vi "FinalProject.vi"() -> ()   [LabVIEW 2016]
uses:
  <vilib>/DAQmx/read.llb/DAQmx Read (Digital Bool 1Line 1Point).vi
  <vilib>/DAQmx/write.llb/DAQmx Write (Digital Bool 1Line 1Point).vi
  <vilib>/DAQmx/create/channels.llb/DAQmx Create Channel (DI-Digital Input).vi
  <vilib>/DAQmx/create/channels.llb/DAQmx Create Channel (DO-Digital Output).vi
  <vilib>/Utility/file.llb/Write Delimited Spreadsheet (DBL).vi
  <vilib>/DAQmx/miscellaneous.llb/DAQmx Fill In Error Info.vi
  <vilib>/ptbypt/NI_PtbyPt.lvlib
panel:
  in  "Stop Button":bool
  in  "Start Button":bool
  out "new file path (Not A Path if cancelled)":path
  out "BELT":bool=TRUE
  out "CHAIN":bool=TRUE
  out "Stop":bool
  out "Start":bool=TRUE
  out "Asem":i32
  out "Temp.1 2":i32
  out "Temp.1":i32
  out "Final Plastic":dbl(slide) scale=0.0..12.0 scale format="%#_12g"
  out "Final Metal":dbl(slide) scale=0.0..12.0 scale format="%#_12g"
  out "Metal detector on QA Rejector":bool
  out "temp.":i32
  out "Final Assembly":i32(knob) scale=0.0..12.0 scale format="%#.12g"
  out "Plastic rejection temp":dbl
  out "Metal rejected temp":dbl
  out "leave assembble":i32
  out "Assembly and Laser":i32
  out "Assembly":i32
  out "Numeric 5":i32
  out "Numeric 4":i32
  in  "stop 2":bool
  out "Assembly Count":u32
  out "Numeric 3":i32
  out "Numeric 2":u32
  out "metal clear 1":u32
  out "Metal Count 2":u32
  out "Metal count temp 2":dbl
  out "Numeric":i32
  out "Assemble Temp":u32
  out "Proximity (BELT)":bool
  in  "QA Rejector (plastic/metal)":bool
  out "Plastic in Chute":dbl(knob) scale=0.0..6.0 scale format="%#_10g"
  out "Metal Detector (CHAIN)":bool
  out "Proximity (CHAIN)":bool
  out "Laser (BELT)":bool
  out "Metal Detector (BELT)":bool
  out "Complete Assembly\n Detector (False when assem is there)":bool
  out "Rotary Proximity":bool
  in  "Rotary Motor":bool
  in  "Kicker (CHAIN)":bool
  in  "stop":bool
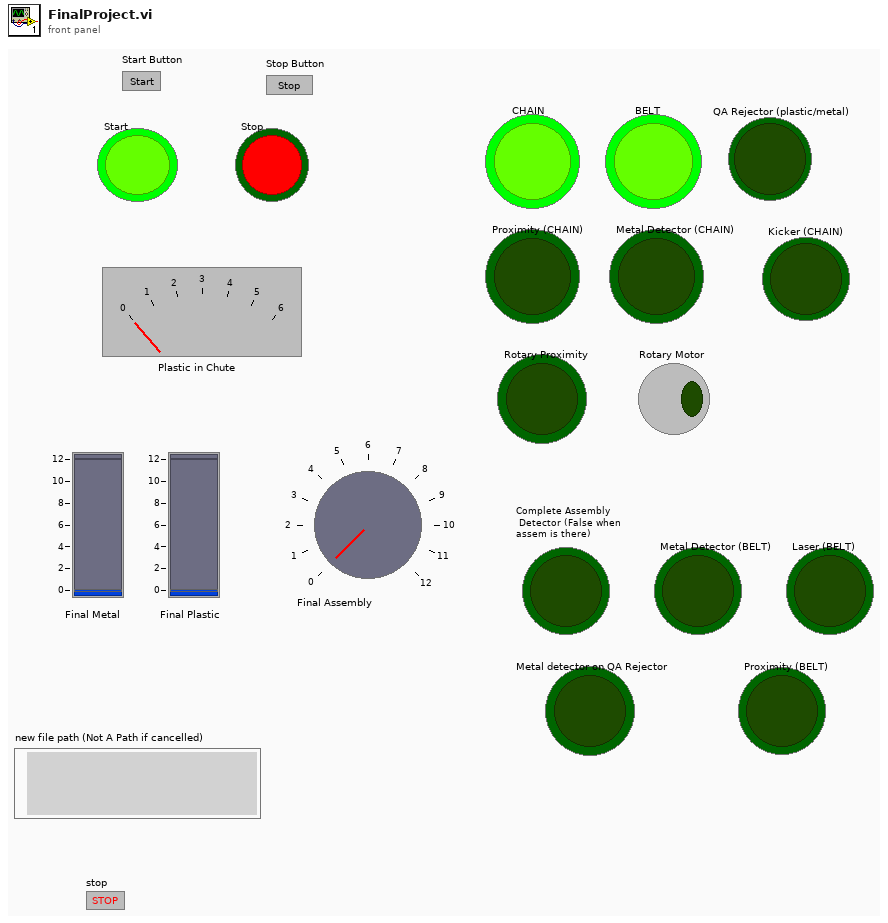
[diagram p1: front panel]
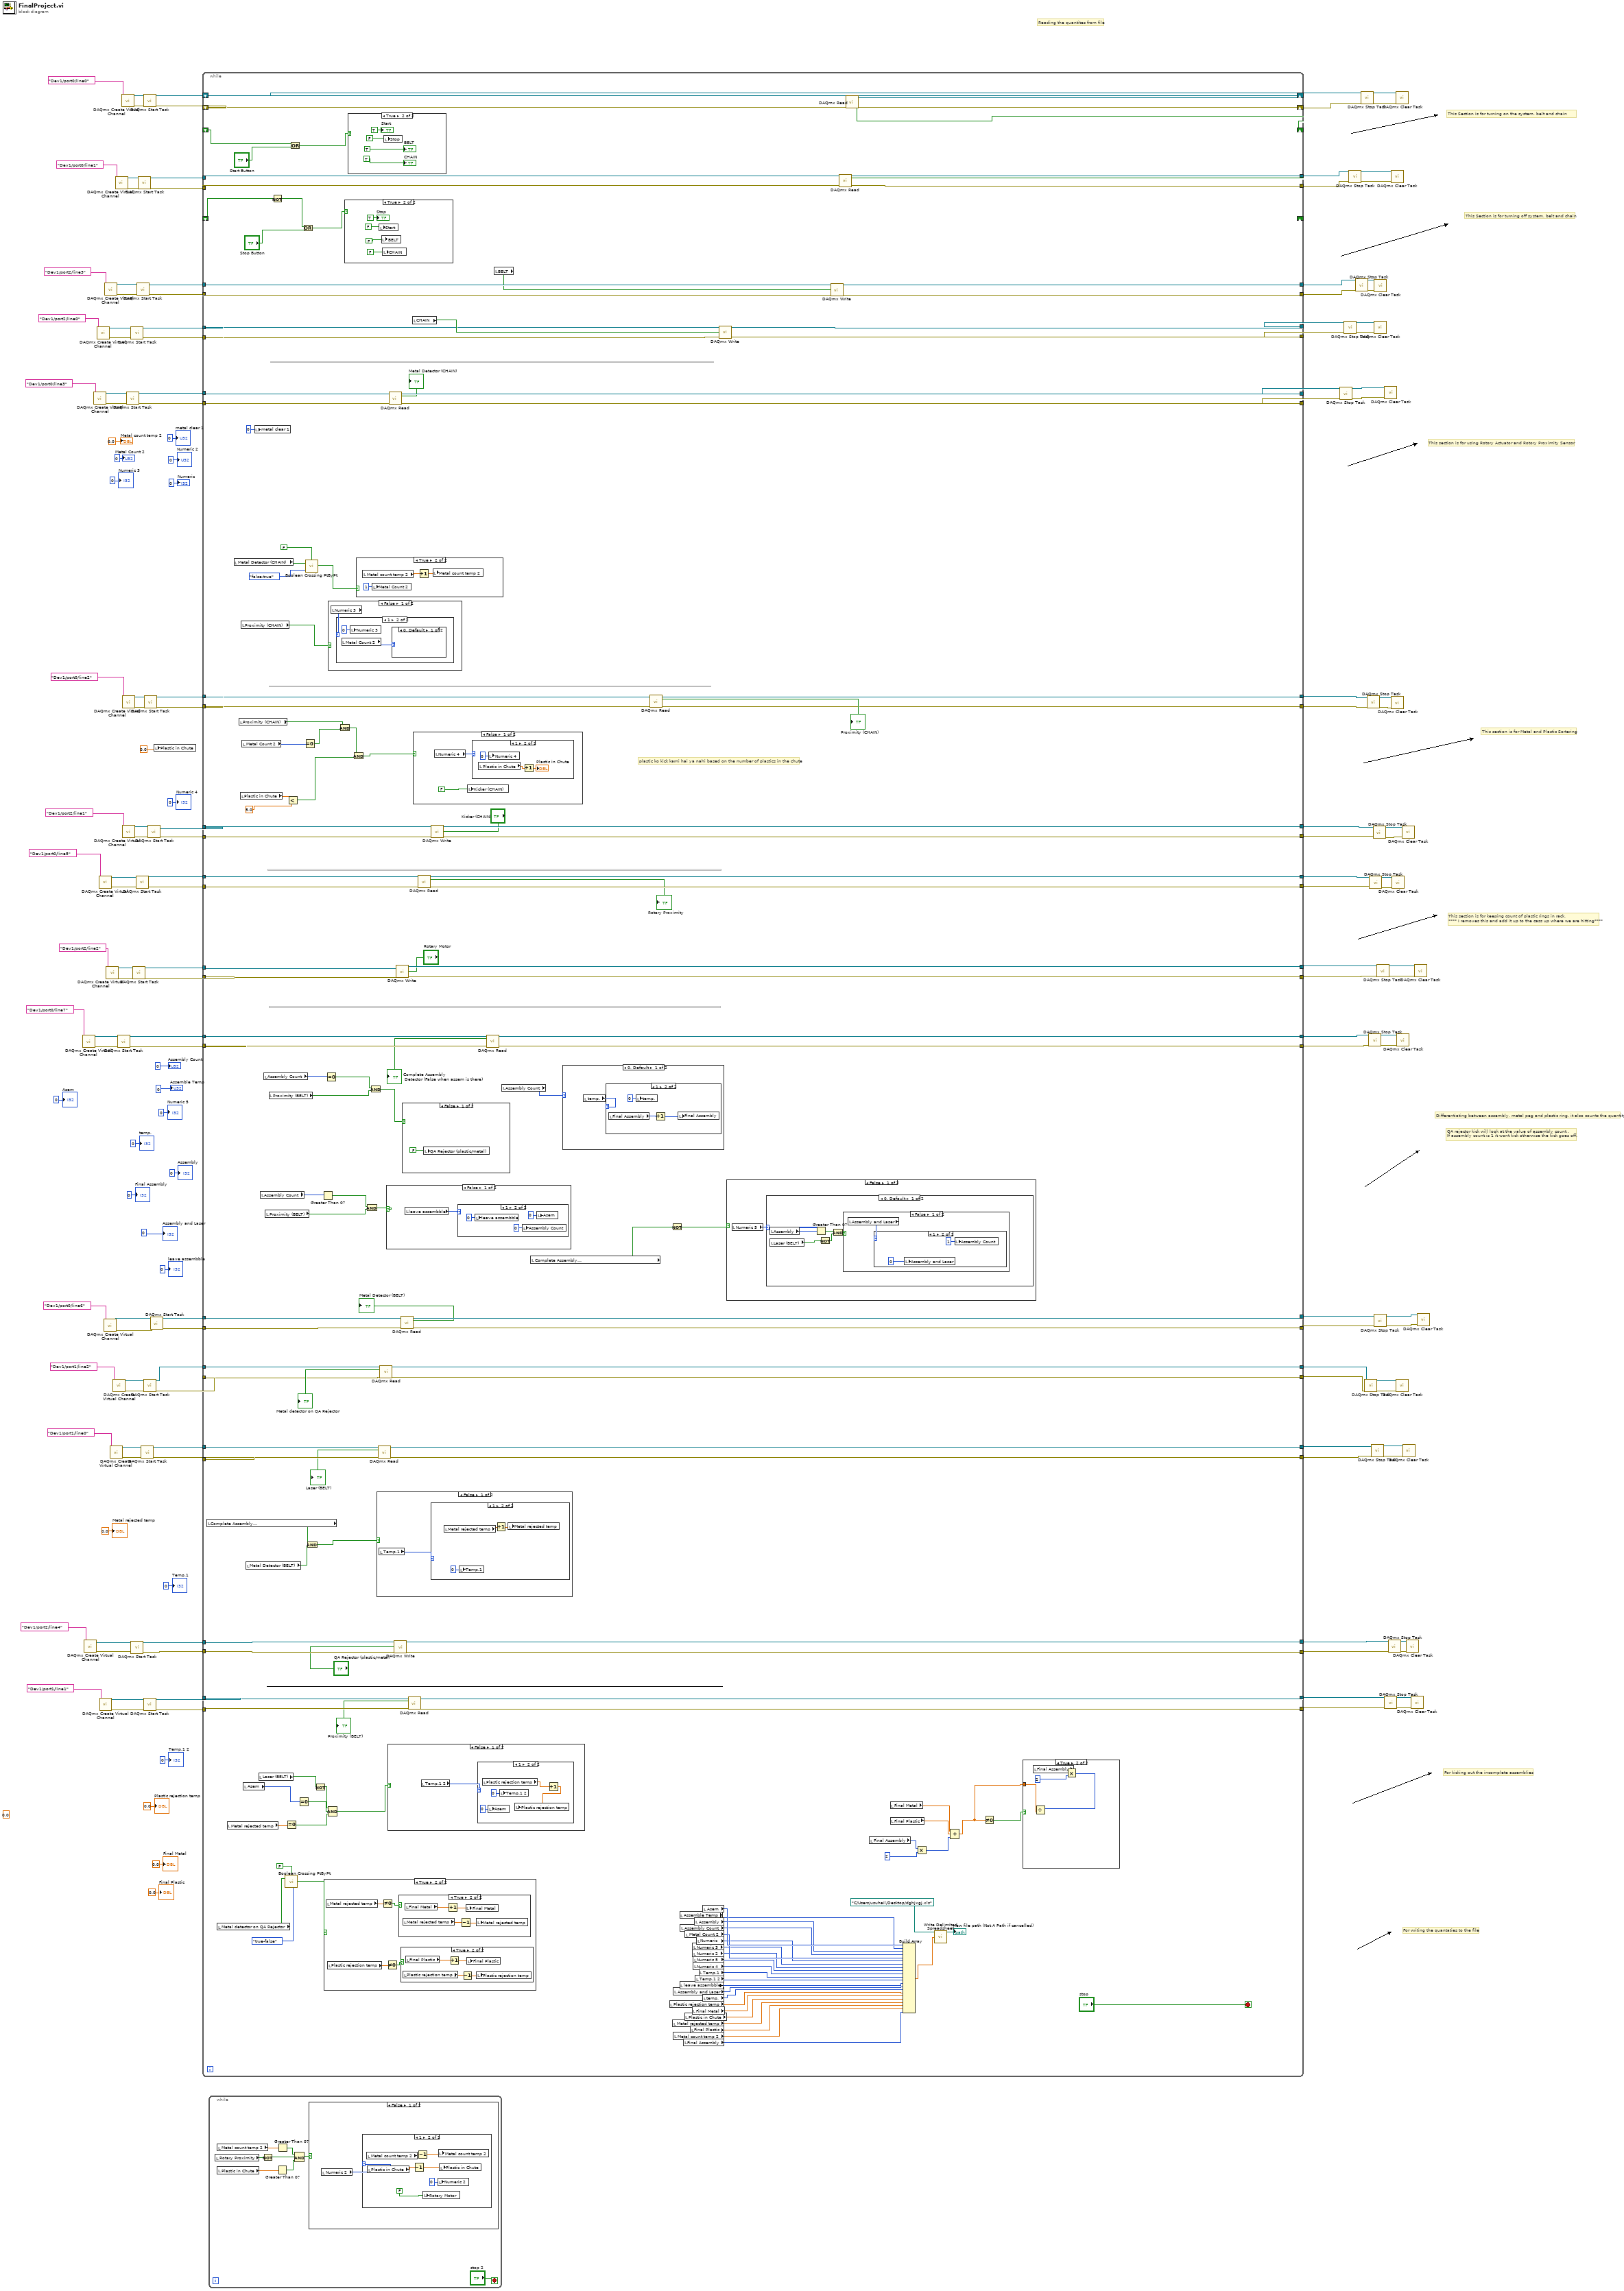
[diagram p0: block diagram]
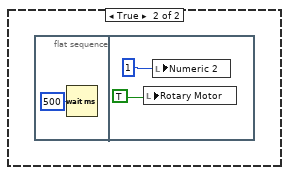
[diagram p3: hidden frame]
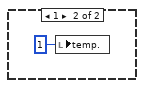
[diagram p9: hidden frame]
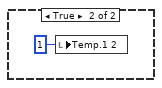
[diagram p11: hidden frame]
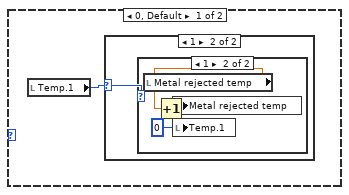
[diagram p12: hidden frame]
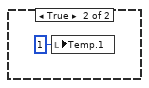
[diagram p15: hidden frame]
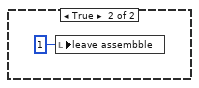
[diagram p17: hidden frame]
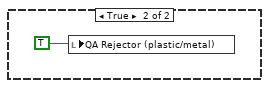
[diagram p18: hidden frame]
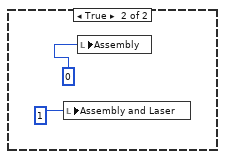
[diagram p20: hidden frame]
diagram:
  (unwired) 0.0
  # "QA rejector kick will look at the value of assembly count .\nIf assembly count is 1 it wont kick otherwise the kick goes off."
  # "Reading the quantites from file"
  # "For writing the quantaties to the file"
  # "For kicking out the incomplete assemblies"
  # "Differentiating between assembly, metal peg and plastic ring. it also counts the quantity"
  # "This section is for keeping count of plastic rings in rack. \n**** I removes this and add it up to the cass up where we are hitting****"
  # "This section is for using Rotory Actuator and Rotory Proximity Sensor"
  # "This Section is for turning off system, belt and chain"
  # "This Section is for turning on the system, belt and chain"
  # "This section is for Metal and Plastic Sortering"
  n1 = call-poly <vilib>:"DAQmx Create Virtual Channel.vi"("lines"=tag "Dev1/port0/line7") -> ("task out"=w76:refnum<k21>, "error out"=w75:errorcluster)  [unwired: 13 in]
  n2 = call-poly <vilib>:"DAQmx Create Virtual Channel.vi"("lines"=tag "Dev1/port2/line4") -> ("task out"=w48:refnum<k21>, "error out"=w47:errorcluster)  [unwired: 13 in]
  n3 = call-poly <vilib>:"DAQmx Create Virtual Channel.vi"("lines"=tag "Dev1/port0/line3") -> ("task out"=w119:refnum<k21>, "error out"=w118:errorcluster)  [unwired: 13 in]
  n4 = call-poly <vilib>:"DAQmx Create Virtual Channel.vi"("lines"=tag "Dev1/port2/line0") -> ("task out"=w128:refnum<k21>, "error out"=w127:errorcluster)  [unwired: 13 in]
  n5 = call-poly <vilib>:"DAQmx Create Virtual Channel.vi"("lines"=tag "Dev1/port0/line5") -> ("task out"=w94:refnum<k21>, "error out"=w93:errorcluster)  [unwired: 13 in]
  n6 = call-poly <vilib>:"DAQmx Create Virtual Channel.vi"("lines"=tag "Dev1/port1/line1") -> ("task out"=w39:refnum<k21>, "error out"=w38:errorcluster)  [unwired: 13 in]
  n7 = call-poly <vilib>:"DAQmx Create Virtual Channel.vi"("lines"=tag "Dev1/port0/line6") -> ("task out"=w69:refnum<k21>, "error out"=w68:errorcluster)  [unwired: 13 in]
  n8 = call-poly <vilib>:"DAQmx Create Virtual Channel.vi"("lines"=tag "Dev1/port2/line3") -> ("task out"=w137:refnum<k21>, "error out"=w136:errorcluster)  [unwired: 13 in]
  n9 = call-poly <vilib>:"DAQmx Create Virtual Channel.vi"("lines"=tag "Dev1/port2/line2") -> ("task out"=w85:refnum<k21>, "error out"=w84:errorcluster)  [unwired: 13 in]
  n10 = call-poly <vilib>:"DAQmx Create Virtual Channel.vi"("lines"=tag "Dev1/port1/line0") -> ("task out"=w58:refnum<k21>, "error out"=w57:errorcluster)  [unwired: 13 in]
  n11 = call-poly <vilib>:"DAQmx Create Virtual Channel.vi"("lines"=tag "Dev1/port1/line2") -> ("task out"=w13:refnum<k21>, "error out"=w14:errorcluster)  [unwired: 13 in]
  n12 = call-poly <vilib>:"DAQmx Create Virtual Channel.vi"("lines"=tag "Dev1/port0/line1") -> ("task out"=w149:refnum<k21>, "error out"=w147:errorcluster)  [unwired: 13 in]
  n13 = call <vilib>:"DAQmx Start Task.vi"("task/channels in"=w76, "error in"=w75) -> ("task out"=w74:refnum<k21>, "error out"=w73:errorcluster)  [unwired: 12 in]
  n14 = call-poly <vilib>:"DAQmx Create Virtual Channel.vi"("lines"=tag "Dev1/port0/line0") -> ("task out"=w158:refnum<k21>, "error out"=w154:errorcluster)  [unwired: 13 in]
  n15 = call-poly <vilib>:"DAQmx Create Virtual Channel.vi"("lines"=tag "Dev1/port0/line2") -> ("task out"=w111:refnum<k21>, "error out"=w110:errorcluster)  [unwired: 13 in]
  n16 = call-poly <vilib>:"DAQmx Create Virtual Channel.vi"("lines"=tag "Dev1/port2/line1") -> ("task out"=w103:refnum<k21>, "error out"=w102:errorcluster)  [unwired: 13 in]
  n17 = call <vilib>:"DAQmx Start Task.vi"("task/channels in"=w119, "error in"=w118) -> ("task out"=w116:refnum<k21>, "error out"=w115:errorcluster)  [unwired: 12 in]
  n18 = call <vilib>:"DAQmx Start Task.vi"("task/channels in"=w128, "error in"=w127) -> ("task out"=w126:refnum<k21>, "error out"=w125:errorcluster)  [unwired: 12 in]
  n19 = call <vilib>:"DAQmx Start Task.vi"("task/channels in"=w48, "error in"=w47) -> ("task out"=w44:refnum<k21>, "error out"=w43:errorcluster)  [unwired: 12 in]
  n20 = call <vilib>:"DAQmx Start Task.vi"("task/channels in"=w85, "error in"=w84) -> ("task out"=w83:refnum<k21>, "error out"=w82:errorcluster)  [unwired: 12 in]
  n21 = call <vilib>:"DAQmx Start Task.vi"("task/channels in"=w94, "error in"=w93) -> ("task out"=w92:refnum<k21>, "error out"=w91:errorcluster)  [unwired: 12 in]
  n22 = call <vilib>:"DAQmx Start Task.vi"("task/channels in"=w137, "error in"=w136) -> ("task out"=w135:refnum<k21>, "error out"=w134:errorcluster)  [unwired: 12 in]
  n23 = call <vilib>:"DAQmx Start Task.vi"("task/channels in"=w149, "error in"=w147) -> ("task out"=w144:refnum<k21>, "error out"=w143:errorcluster)  [unwired: 12 in]
  n24 = call <vilib>:"DAQmx Start Task.vi"("task/channels in"=w58, "error in"=w57) -> ("task out"=w56:refnum<k21>, "error out"=w55:errorcluster)  [unwired: 12 in]
  n25 = call <vilib>:"DAQmx Start Task.vi"("task/channels in"=w158, "error in"=w154) -> ("task out"=w157:refnum<k21>, "error out"=w153:errorcluster)  [unwired: 12 in]
  n26 = call <vilib>:"DAQmx Start Task.vi"("task/channels in"=w39, "error in"=w38) -> ("task out"=w37:refnum<k21>, "error out"=w36:errorcluster)  [unwired: 12 in]
  n27 = call <vilib>:"DAQmx Start Task.vi"("task/channels in"=w13, "error in"=w14) -> ("task out"=w11:refnum<k21>, "error out"=w10:errorcluster)  [unwired: 12 in]
  n28 = call <vilib>:"DAQmx Start Task.vi"("task/channels in"=w111, "error in"=w110) -> ("task out"=w109:refnum<k21>, "error out"=w108:errorcluster)  [unwired: 12 in]
  n29 = call <vilib>:"DAQmx Start Task.vi"("task/channels in"=w103, "error in"=w102) -> ("task out"=w101:refnum<k21>, "error out"=w100:errorcluster)  [unwired: 12 in]
  n30 = call <vilib>:"DAQmx Start Task.vi"("task/channels in"=w69, "error in"=w68) -> ("task out"=w65:refnum<k21>, "error out"=w60:errorcluster)  [unwired: 12 in]
  n31 = local write "Plastic in Chute"(0.0) -> ()
  n32 = while {
    shift-right: [w311] -> w156
    shift-left: w157 -> [w312]
    shift-right: [w309] -> w152
    shift-left: w153 -> [w310]
    shift-right: [w307] -> _
    shift-left: _ -> [w164]
    tunnel: w144 -> [w306]
    tunnel: w143 -> [w305]
    tunnel: [w304] -> w142
    tunnel: [w303] -> w141
    shift-right: [w302] -> _
    shift-left: _ -> [w301]
    tunnel: w135 -> [w297]
    tunnel: w134 -> [w300]
    tunnel: [w299] -> w133
    tunnel: [w298] -> w132
    tunnel: w126 -> [w293]
    tunnel: w125 -> [w294]
    tunnel: [w292] -> w124
    tunnel: [w291] -> w123
    tunnel: [w285] -> w117
    tunnel: w116 -> [w287]
    tunnel: w115 -> [w286]
    tunnel: w109 -> [w290]
    tunnel: w108 -> [w289]
    tunnel: [w288] -> w106
    tunnel: [w228] -> w107
    tunnel: [w231] -> w105
    tunnel: w101 -> [w284]
    tunnel: w100 -> [w283]
    tunnel: [w282] -> w99
    tunnel: [w281] -> w98
    tunnel: w92 -> [w280]
    tunnel: w91 -> [w279]
    tunnel: [w278] -> w88
    tunnel: [w277] -> w87
    tunnel: w83 -> [w276]
    tunnel: w82 -> [w275]
    tunnel: [w274] -> w79
    tunnel: [w273] -> w78
    tunnel: w74 -> [w271]
    tunnel: w73 -> [w268]
    tunnel: w65 -> [w267]
    tunnel: [w265] -> w64
    tunnel: [w264] -> w63
    tunnel: [w270] -> w62
    tunnel: [w269] -> w61
    tunnel: w60 -> [w266]
    tunnel: w56 -> [w259]
    tunnel: w55 -> [w258]
    tunnel: [w257] -> w52
    tunnel: [w256] -> w51
    tunnel: w44 -> [w243]
    tunnel: w43 -> [w240]
    tunnel: [w242] -> w42
    tunnel: [w241] -> w41
    tunnel: w37 -> [w238]
    tunnel: w36 -> [w237]
    tunnel: [w236] -> w33
    tunnel: [w235] -> w32
    tunnel: w11 -> [w214]
    tunnel: w10 -> [w213]
    tunnel: [w212] -> w7
    tunnel: [w211] -> w6
    stop <- "stop" stop-if-true
    # "plastic ko kick karni hai ya nahi based on the number of plastics in the chute"
    n33 = local read "Complete Assembly\n Detector (False when assem is there)"() -> (w206:bool)
    n34 = local read "Metal detector on QA Rejector"() -> (w209:bool)
    n35 = local read "Metal rejected temp"() -> (w203:dbl)
    n36 = local read "Metal Detector (CHAIN)"() -> (w233:bool)
    n37 = local read "Proximity (CHAIN)"() -> (w250:bool)
    n38 = local read "Plastic in Chute"() -> (w247:dbl)
    n39 = local read "Proximity (CHAIN)"() -> (w229:bool)
    n40 = local read "Metal Count 2"() -> (w230:u32)
    n41 = local read "Asem"() -> (w197:i32)
    n42 = local read "Metal Detector (BELT)"() -> (w205:bool)
    n43 = local write "metal clear 1"(u32 0 ("metal clear 1")) -> ()
    n44 = local read "Laser (BELT)"() -> (w201:bool)
    n45 = local read "Assembly Count"() -> (w219:u32)
    n46 = local read "Assembly Count"() -> (w226:u32)
    n47 = local read "Proximity (BELT)"() -> (w221:bool)
    n48 = local read "Proximity (BELT)"() -> (w224:bool)
    n49 = Not(x=w301) -> (.not. x?=w160:bool)
    n50 = call <vilib>:"Boolean Crossing PtByPt.vi"("initialize"=FALSE, "direction"=enum16{"either", "false-true", "true-false"}."true-false", "input"=w209) -> ("crossing"=w208:bool)
    n51 = Equal To 0?(x=w203) -> (x = 0?=w202:bool)
    n52 = Less?(x=w247, y=5.0) -> (x < y?=w244:bool)
    n53 = Or(x=w164, y="Start Button") -> (x .or. y?=w162:bool)
    n54 = Equal To 0?(x=w197) -> (x = 0?=w199:bool)
    n55 = Or(x=w160, y="Stop Button") -> (x .or. y?=w159:bool)
    n56 = Equal To 0?(x=w230) -> (x = 0?=w249:bool)
    n57 = call <vilib>:"Boolean Crossing PtByPt.vi"("initialize"=FALSE, "direction"=enum16{"either", "false-true", "true-false"}."false-true", "input"=w233) -> ("crossing"=w251:bool)
    n58 = And(x=w206, y=w205) -> (x .and. y?=w204:bool)
    n59 = Not(x=w201) -> (.not. x?=w200:bool)
    n60 = Greater Than 0?(x=w219) -> (x > 0?=w220:bool)
    n61 = case shown="True" w208 {
      frame False {
      }
      frame True {
        n62 = local read "Metal rejected temp"() -> (w320:dbl)
        n63 = local read "Plastic rejection temp"() -> (w318:dbl)
        n64 = Not Equal To 0?(x=w320) -> (x != 0?=w319:bool)
        n65 = Not Equal To 0?(x=w318) -> (x != 0?=w317:bool)
        n66 = case shown="True" w319 {
          frame False {
          }
          frame True {
            n67 = local read "Metal rejected temp"() -> (w326:dbl)
            n68 = local read "Final Metal"() -> (w327:dbl)
            n69 = Increment(x=w327) -> (x+1=w328:dbl)
            n70 = Decrement(x=w326) -> (x-1=w325:dbl)
            n71 = local write "Final Metal"(w328) -> ()
            n72 = local write "Metal rejected temp"(w325) -> ()
          }
        }
        n73 = case shown="True" w317 {
          frame False {
          }
          frame True {
            n74 = local read "Plastic rejection temp"() -> (w323:dbl)
            n75 = local read "Final Plastic"() -> (w322:dbl)
            n76 = Increment(x=w322) -> (x+1=w321:dbl)
            n77 = Decrement(x=w323) -> (x-1=w324:dbl)
            n78 = local write "Final Plastic"(w321) -> ()
            n79 = local write "Plastic rejection temp"(w324) -> ()
          }
        }
      }
    }
    n80 = Equal To 0?(x=w226) -> (x = 0?=w225:bool)
    n81 = case shown="False" w229 {
      frame False {
        n82 = local read "Numeric 3"() -> (w372:i32)
        n83 = case shown="1" w372 {
          frame 0, Default {
          }
          frame 1 {
            n84 = local read "Metal Count 2"() -> (w373:u32)
            n85 = local write "Numeric 3"(0 ("Numeric 3")) -> ()
            n86 = case shown="0, Default" w373 {
              frame 0, Default {
              }
              frame 1 {
                n87 = local write "Metal Count 2"(u32 0 ("Metal Count 2")) -> ()
              }
            }
          }
        }
      }
      frame True {
        n88 = local write "Numeric 3"(1 ("Numeric 3")) -> ()
      }
    }
    n89 = Compound Arithmetic op=AND(w200, w199, w202) -> (w198:bool)
    n90 = And(x=w250, y=w249) -> (x .and. y?=w245:bool)
    n91 = case shown="True" w159 {
      frame False {
      }
      frame True {
        n92 = local write "Start"(FALSE) -> ()
        n93 = local write "BELT"(FALSE) -> ()
        n94 = local write "CHAIN"(FALSE) -> ()
        "Stop" <- TRUE
      }
    }
    n95 = case shown="True" w162 {
      frame False {
      }
      frame True {
        n96 = local write "Stop"(FALSE) -> ()
        "Start" <- TRUE
        "BELT" <- TRUE
        "CHAIN" <- TRUE
      }
    }
    n97 = And(x=w245, y=w244) -> (x .and. y?=w246:bool)
    n98 = case shown="True" w251 {
      frame False {
      }
      frame True {
        n99 = local read "Metal count temp 2"() -> (w379:dbl)
        n100 = local write "Metal Count 2"(u32 1 ("Metal Count 2")) -> ()
        n101 = Increment(x=w379) -> (x+1=w378:dbl)
        n102 = local write "Metal count temp 2"(w378) -> ()
      }
    }
    n103 = And(x=w220, y=w221) -> (x .and. y?=w222:bool)
    n104 = And(x=w225, y=w224) -> (x .and. y?=w223:bool)
    n105 = case shown="False" w204 {
      frame False {
        n106 = local read "Temp.1"() -> (w340:i32)
        n107 = case shown="1" w340 {
          frame 0, Default {
            n108 = local read "Temp.1"() -> (w341:i32)
            n109 = case shown="1" w341 {
              selector: w341 -> [_ w342]
              frame 0, Default {
              }
              frame 1 {
                n110 = case shown="1" w342 {
                  frame 0, Default {
                  }
                  frame 1 {
                    n111 = local read "Metal rejected temp"() -> (w343:dbl)
                    n112 = Increment(x=w343) -> (x+1=w344:dbl)
                    n113 = local write "Metal rejected temp"(w344) -> ()
                    n114 = local write "Temp.1"(0 ("Temp.1")) -> ()
                  }
                }
              }
            }
          }
          frame 1 {
            n115 = local read "Metal rejected temp"() -> (w347:dbl)
            n116 = local write "Temp.1"(0 ("Temp.1")) -> ()
            n117 = Increment(x=w347) -> (x+1=w346:dbl)
            n118 = local write "Metal rejected temp"(w346) -> ()
          }
        }
      }
      frame True {
        n119 = local write "Temp.1"(1 ("Temp.1")) -> ()
      }
    }
    n120 = call-poly <vilib>:"DAQmx Read.vi"("task/channels in"=w259, "error in"=w258) -> ("task out"=w257:refnum<k21>, "data"=→"Laser (BELT)":bool, "error out"=w256:errorcluster)  [unwired: 11 in]
    n121 = call-poly <vilib>:"DAQmx Read.vi"("task/channels in"=w214, "error in"=w213) -> ("task out"=w211:refnum<k21>, "data"=→"Metal detector on QA Rejector":bool, "error out"=w212:errorcluster)  [unwired: 11 in]
    n122 = case shown="False" w222 {
      frame False {
        n123 = local read "leave assembble"() -> (w350:i32)
        n124 = case shown="1" w350 {
          frame 0, Default {
          }
          frame 1 {
            n125 = local write "leave assembble"(0 ("leave assembble")) -> ()
            n126 = local write "Assembly Count"(u32 0 ("Assembly Count")) -> ()
            n127 = local write "Asem"(0 ("Asem")) -> ()
          }
        }
      }
      frame True {
        n128 = local write "leave assembble"(1 ("leave assembble")) -> ()
      }
    }
    n129 = case shown="False" w198 {
      frame False {
        n130 = local read "Temp.1 2"() -> (w334:i32)
        n131 = case shown="1" w334 {
          frame 0, Default {
          }
          frame 1 {
            n132 = local read "Plastic rejection temp"() -> (w338:dbl)
            n133 = local write "Asem"(0 ("Asem")) -> ()
            n134 = local write "Temp.1 2"(0 ("Temp.1 2")) -> ()
            n135 = Increment(x=w338) -> (x+1=w337:dbl)
            n136 = local write "Plastic rejection temp"(w337) -> ()
          }
        }
      }
      frame True {
        n137 = local write "Temp.1 2"(1 ("Temp.1 2")) -> ()
      }
    }
    n138 = call-poly <vilib>:"DAQmx Read.vi"("task/channels in"=w287, "error in"=w286) -> ("task out"=w285:refnum<k21>, "data"=→"Metal Detector (CHAIN)":bool, "error out"=w231:errorcluster)  [unwired: 11 in]
    n139 = call-poly <vilib>:"DAQmx Write.vi"("task/channels in"=w243, "data"="QA Rejector (plastic/metal)", "error in"=w240) -> ("task out"=w242:refnum<k21>, "error out"=w241:errorcluster)  [unwired: 10 in, 1 out]
    n140 = call-poly <vilib>:"DAQmx Write.vi"("task/channels in"=w276, "data"="Rotary Motor", "error in"=w275) -> ("task out"=w274:refnum<k21>, "error out"=w273:errorcluster)  [unwired: 10 in, 1 out]
    n141 = call-poly <vilib>:"DAQmx Read.vi"("task/channels in"=w267, "error in"=w266) -> ("task out"=w265:refnum<k21>, "data"=→"Metal Detector (BELT)":bool, "error out"=w264:errorcluster)  [unwired: 11 in]
    n142 = case shown="False" w223 {
      frame False {
        n143 = local write "QA Rejector (plastic/metal)"(FALSE ("Solinoid(polo or metal rejector) 2")) -> ()
      }
      frame True {
        n144 = local write "QA Rejector (plastic/metal)"(TRUE ("Solinoid(polo or metal rejector) 2")) -> ()
      }
    }
    n145 = call-poly <vilib>:"DAQmx Read.vi"("task/channels in"=w238, "error in"=w237) -> ("task out"=w236:refnum<k21>, "data"=→"Proximity (BELT)":bool, "error out"=w235:errorcluster)  [unwired: 11 in]
    n146 = local read "CHAIN"() -> (w295:bool)
    n147 = case shown="False" w246 {
      frame False {
        n148 = local read "Numeric 4"() -> (w380:i32)
        n149 = local write "Kicker (CHAIN)"(FALSE) -> ()
        n150 = case shown="1" w380 {
          frame 0, Default {
          }
          frame 1 {
            n151 = local read "Plastic in Chute"() -> (w382:dbl)
            n152 = local write "Numeric 4"(0 ("Numeric 4")) -> ()
            n153 = Increment(x=w382) -> (x+1=→"Plastic in Chute":dbl)
          }
        }
      }
      frame True {
        n154 = local write "Kicker (CHAIN)"(TRUE) -> ()
        n155 = local write "Numeric 4"(1 ("Numeric 4")) -> ()
      }
    }
    n156 = call-poly <vilib>:"DAQmx Read.vi"("task/channels in"=w280, "error in"=w279) -> ("task out"=w278:refnum<k21>, "data"=→"Rotary Proximity":bool, "error out"=w277:errorcluster)  [unwired: 11 in]
    n157 = call-poly <vilib>:"DAQmx Write.vi"("task/channels in"=w284, "data"="Kicker (CHAIN)", "error in"=w283) -> ("task out"=w282:refnum<k21>, "error out"=w281:errorcluster)  [unwired: 10 in, 1 out]
    n158 = call-poly <vilib>:"DAQmx Read.vi"("task/channels in"=w271, "error in"=w268) -> ("task out"=w269:refnum<k21>, "data"=→"Complete Assembly\n Detector (False when assem is there)":bool, "error out"=w270:errorcluster)  [unwired: 11 in]
    n159 = local read "BELT"() -> (w296:bool)
    n160 = local read "Assembly Count"() -> (w216:u32)
    n161 = local read "Complete Assembly\n Detector (False when assem is there)"() -> (w218:bool)
    n162 = case shown="0, Default" w216 {
      frame 0, Default {
        n163 = local read "temp."() -> (w329:i32)
        n164 = case shown="1" w329 {
          frame 0, Default {
          }
          frame 1 {
            n165 = local read "Final Assembly"() -> (w331:i32)
            n166 = local write "temp."(0 ("temp.")) -> ()
            n167 = Increment(x=w331) -> (x+1=w330:i32)
            n168 = local write "Final Assembly"(w330) -> ()
          }
        }
      }
      frame 1 {
        n169 = local write "temp."(1 ("temp.")) -> ()
      }
    }
    n170 = call-poly <vilib>:"DAQmx Read.vi"("task/channels in"=w290, "error in"=w289) -> ("task out"=w288:refnum<k21>, "data"=→"Proximity (CHAIN)":bool, "error out"=w228:errorcluster)  [unwired: 11 in]
    n171 = local read "Plastic rejection temp"() -> (w171:dbl)
    n172 = Not(x=w218) -> (.not. x?=w217:bool)
    n173 = local read "Metal rejected temp"() -> (w168:dbl)
    n174 = local read "Assembly and Laser"() -> (w173:i32)
    n175 = local read "Metal count temp 2"() -> (w166:dbl)
    n176 = local read "Assemble Temp"() -> (w185:u32)
    n177 = local read "leave assembble"() -> (w174:i32)
    n178 = local read "Assembly Count"() -> (w183:u32)
    n179 = local read "Final Assembly"() -> (w165:i32)
    n180 = local read "Plastic in Chute"() -> (w169:dbl)
    n181 = local read "Metal Count 2"() -> (w182:u32)
    n182 = local read "Final Plastic"() -> (w167:dbl)
    n183 = local read "Final Metal"() -> (w170:dbl)
    n184 = local read "Numeric 3"() -> (w180:i32)
    n185 = local read "Numeric 2"() -> (w179:u32)
    n186 = local read "Numeric 5"() -> (w178:i32)
    n187 = local read "Numeric 4"() -> (w177:i32)
    n188 = local read "Assembly"() -> (w184:i32)
    n189 = local read "Temp.1 2"() -> (w175:i32)
    n190 = local read "Numeric"() -> (w181:i32)
    n191 = local read "Temp.1"() -> (w176:i32)
    n192 = local read "temp."() -> (w172:i32)
    n193 = local read "Asem"() -> (w186:i32)
    n194 = call-poly <vilib>:"DAQmx Write.vi"("task/channels in"=w293, "data"=w295, "error in"=w294) -> ("task out"=w292:refnum<k21>, "error out"=w291:errorcluster)  [unwired: 10 in, 1 out]
    n195 = case shown="False" w217 {
      frame False {
        n196 = local read "Numeric 5"() -> (w357:i32)
        n197 = case shown="0, Default" w357 {
          frame 0, Default {
            n198 = local read "Assembly"() -> (w360:i32)
            n199 = local read "Laser (BELT)"() -> (w362:bool)
            n200 = Greater Than 0?(x=w360) -> (x > 0?=w359:bool)
            n201 = Not(x=w362) -> (.not. x?=w358:bool)
            n202 = And(x=w359, y=w358) -> (x .and. y?=w361:bool)
            n203 = case shown="False" w361 {
              frame False {
                n204 = local read "Assembly and Laser"() -> (w363:i32)
                n205 = case shown="1" w363 {
                  frame 0, Default {
                  }
                  frame 1 {
                    n206 = local write "Assembly and Laser"(0 ("Assembly and Laser")) -> ()
                    n207 = local write "Assembly Count"(u32 1 ("Assembly Count")) -> ()
                  }
                }
              }
              frame True {
                n208 = local write "Assembly and Laser"(1 ("Assembly and Laser")) -> ()
                n209 = local write "Assembly"(0 ("Assembly")) -> ()
              }
            }
          }
          frame 1 {
            n210 = local write "Numeric 5"(0 ("Numeric 5")) -> ()
            n211 = local write "Assembly"(1 ("Assembly")) -> ()
          }
        }
      }
      frame True {
        n212 = local write "Numeric 5"(1 ("Numeric 5")) -> ()
        n213 = local write "Asem"(1 ("Asem")) -> ()
      }
    }
    n214 = call-poly <vilib>:"DAQmx Write.vi"("task/channels in"=w297, "data"=w296, "error in"=w300) -> ("task out"=w298:refnum<k21>, "error out"=w299:errorcluster)  [unwired: 10 in, 1 out]
    n215 = call-poly <vilib>:"DAQmx Read.vi"("task/channels in"=w306, "error in"=w305) -> ("task out"=w304:refnum<k21>, "data"=w302:bool, "error out"=w303:errorcluster)  [unwired: 11 in]
    n216 = call-poly <vilib>:"DAQmx Read.vi"("task/channels in"=w312, "error in"=w310) -> ("task out"=w311:refnum<k21>, "data"=w307:bool, "error out"=w309:errorcluster)  [unwired: 11 in]
    n217 = local read "Final Assembly"() -> (w195:i32)
    n218 = local read "Final Metal"() -> (w192:dbl)
    n219 = local read "Final Plastic"() -> (w193:dbl)
    n220 = Build Array(w186, w185, w184, w183, w182, w181, w180, w179, w178, w177, w176, w175, w174, w173, w172, w171, w170, w169, w168, w167, w166, w165) -> (w189:dbl[])
    n221 = Multiply(x=w195, y=2) -> (x*y=w194:i32)
    n222 = call-poly <vilib>:"Write Delimited Spreadsheet.vi"("file path (dialog if empty)"=path "C:/Users/usuhail/Desktop/dghjxgj.xls", "1D data"=w189) -> ("new file path (Not A Path if cancelled)"=→"new file path (Not A Path if cancelled)":path)  [unwired: 12 in, 1 out]
    n223 = Compound Arithmetic op=ADD(w192, w193, w194) -> (w190:dbl)
    n224 = Not Equal To 0?(x=w190) -> (x != 0?=w191:bool)
    n225 = case shown="True" w191 {
      tunnel: w190 -> [_ w313]
      frame False {
      }
      frame True {
        n226 = local read "Final Assembly"() -> (w316:i32)
        n227 = Multiply(x=w316, y=2) -> (x*y=w314:i32)
        n228 = Divide(x=w314, y=w313) -> ()  [unwired: 1 out]
      }
    }
  }
  n229 = while {
    stop <- "stop 2" stop-if-true
    n230 = local read "Rotary Proximity"() -> (w396:bool)
    n231 = local read "Metal count temp 2"() -> (w400:dbl)
    n232 = local read "Plastic in Chute"() -> (w401:dbl)
    n233 = Not(x=w396) -> (.not. x?=w398:bool)
    n234 = Greater Than 0?(x=w401) -> (x > 0?=w402:bool)
    n235 = Greater Than 0?(x=w400) -> (x > 0?=w397:bool)
    n236 = Compound Arithmetic op=AND(w397, w398, w402) -> (w399:bool)
    n237 = case shown="False" w399 {
      frame False {
        n238 = local read "Numeric 2"() -> (w403:u32)
        n239 = case shown="1" w403 {
          frame 0, Default {
          }
          frame 1 {
            n240 = local read "Metal count temp 2"() -> (w407:dbl)
            n241 = local read "Plastic in Chute"() -> (w408:dbl)
            n242 = Decrement(x=w408) -> (x-1=w409:dbl)
            n243 = Decrement(x=w407) -> (x-1=w406:dbl)
            n244 = local write "Rotary Motor"(FALSE) -> ()
            n245 = local write "Numeric 2"(u32 0 ("Numeric 2")) -> ()
            n246 = local write "Metal count temp 2"(w406) -> ()
            n247 = local write "Plastic in Chute"(w409) -> ()
          }
        }
      }
      frame True {
        n248 = flat-sequence {
          frame #0 {
            n249 = Wait (ms)(milliseconds to wait=u32 500) -> ()  [unwired: 1 out]
          }
          frame #1 {
            n250 = local write "Rotary Motor"(TRUE) -> ()
            n251 = local write "Numeric 2"(u32 1) -> ()
          }
        }
      }
    }
  }
  n252 = call <vilib>:"DAQmx Stop Task.vi"("task/channels in"=w117, "error in"=w105) -> ("task out"=w122:refnum<k21>, "error out"=w121:errorcluster)  [unwired: 12 in]
  n253 = call <vilib>:"DAQmx Stop Task.vi"("task/channels in"=w124, "error in"=w123) -> ("task out"=w131:refnum<k21>, "error out"=w130:errorcluster)  [unwired: 12 in]
  n254 = call <vilib>:"DAQmx Stop Task.vi"("task/channels in"=w142, "error in"=w141) -> ("task out"=w148:refnum<k21>, "error out"=w146:errorcluster)  [unwired: 12 in]
  n255 = call <vilib>:"DAQmx Stop Task.vi"("task/channels in"=w132, "error in"=w133) -> ("task out"=w139:refnum<k21>, "error out"=w138:errorcluster)  [unwired: 12 in]
  n256 = call <vilib>:"DAQmx Stop Task.vi"("task/channels in"=w156, "error in"=w152) -> ("task out"=w155:refnum<k21>, "error out"=w151:errorcluster)  [unwired: 12 in]
  n257 = call <vilib>:"DAQmx Stop Task.vi"("task/channels in"=w6, "error in"=w7) -> ("task out"=w8:refnum<k21>, "error out"=w9:errorcluster)  [unwired: 12 in]
  n258 = call <vilib>:"DAQmx Stop Task.vi"("task/channels in"=w106, "error in"=w107) -> ("task out"=w114:refnum<k21>, "error out"=w113:errorcluster)  [unwired: 12 in]
  n259 = call <vilib>:"DAQmx Stop Task.vi"("task/channels in"=w61, "error in"=w62) -> ("task out"=w72:refnum<k21>, "error out"=w71:errorcluster)  [unwired: 12 in]
  n260 = call <vilib>:"DAQmx Stop Task.vi"("task/channels in"=w88, "error in"=w87) -> ("task out"=w90:refnum<k21>, "error out"=w89:errorcluster)  [unwired: 12 in]
  n261 = call <vilib>:"DAQmx Stop Task.vi"("task/channels in"=w52, "error in"=w51) -> ("task out"=w54:refnum<k21>, "error out"=w53:errorcluster)  [unwired: 12 in]
  n262 = call <vilib>:"DAQmx Stop Task.vi"("task/channels in"=w99, "error in"=w98) -> ("task out"=w97:refnum<k21>, "error out"=w96:errorcluster)  [unwired: 12 in]
  n263 = call <vilib>:"DAQmx Clear Task.vi"("task in"=w131, "error in"=w130) -> ()  [unwired: 13 in, 1 out]
  n264 = call <vilib>:"DAQmx Stop Task.vi"("task/channels in"=w64, "error in"=w63) -> ("task out"=w67:refnum<k21>, "error out"=w66:errorcluster)  [unwired: 12 in]
  n265 = call <vilib>:"DAQmx Clear Task.vi"("task in"=w139, "error in"=w138) -> ()  [unwired: 13 in, 1 out]
  n266 = call <vilib>:"DAQmx Stop Task.vi"("task/channels in"=w79, "error in"=w78) -> ("task out"=w81:refnum<k21>, "error out"=w80:errorcluster)  [unwired: 12 in]
  n267 = call <vilib>:"DAQmx Clear Task.vi"("task in"=w122, "error in"=w121) -> ()  [unwired: 13 in, 1 out]
  n268 = call <vilib>:"DAQmx Stop Task.vi"("task/channels in"=w33, "error in"=w32) -> ("task out"=w35:refnum<k21>, "error out"=w34:errorcluster)  [unwired: 12 in]
  n269 = call <vilib>:"DAQmx Stop Task.vi"("task/channels in"=w42, "error in"=w41) -> ("task out"=w46:refnum<k21>, "error out"=w45:errorcluster)  [unwired: 12 in]
  n270 = call <vilib>:"DAQmx Clear Task.vi"("task in"=w148, "error in"=w146) -> ()  [unwired: 13 in, 1 out]
  n271 = call <vilib>:"DAQmx Clear Task.vi"("task in"=w114, "error in"=w113) -> ()  [unwired: 13 in, 1 out]
  n272 = call <vilib>:"DAQmx Clear Task.vi"("task in"=w90, "error in"=w89) -> ()  [unwired: 13 in, 1 out]
  n273 = call <vilib>:"DAQmx Clear Task.vi"("task in"=w155, "error in"=w151) -> ()  [unwired: 13 in, 1 out]
  n274 = call <vilib>:"DAQmx Clear Task.vi"("task in"=w8, "error in"=w9) -> ()  [unwired: 13 in, 1 out]
  n275 = call <vilib>:"DAQmx Clear Task.vi"("task in"=w72, "error in"=w71) -> ()  [unwired: 13 in, 1 out]
  n276 = call <vilib>:"DAQmx Clear Task.vi"("task in"=w97, "error in"=w96) -> ()  [unwired: 13 in, 1 out]
  n277 = call <vilib>:"DAQmx Clear Task.vi"("task in"=w54, "error in"=w53) -> ()  [unwired: 13 in, 1 out]
  n278 = call <vilib>:"DAQmx Clear Task.vi"("task in"=w46, "error in"=w45) -> ()  [unwired: 13 in, 1 out]
  n279 = call <vilib>:"DAQmx Clear Task.vi"("task in"=w35, "error in"=w34) -> ()  [unwired: 13 in, 1 out]
  n280 = call <vilib>:"DAQmx Clear Task.vi"("task in"=w81, "error in"=w80) -> ()  [unwired: 13 in, 1 out]
  n281 = call <vilib>:"DAQmx Clear Task.vi"("task in"=w67, "error in"=w66) -> ()  [unwired: 13 in, 1 out]
  "Assemble Temp" <- u32 0
  "Numeric" <- 0
  "Metal Count 2" <- u32 0 ("Metal Count 2")
  "Metal count temp 2" <- 0.0 ("Metal count temp 2")
  "metal clear 1" <- u32 0 ("Numeric 2")
  "Numeric 2" <- u32 0 ("Numeric 2")
  "Numeric 3" <- 0 ("Numeric 3")
  "Assembly Count" <- u32 0 ("Assembly temp")
  "Numeric 4" <- 0
  "Numeric 5" <- 0
  "Assembly" <- 0
  "Assembly and Laser" <- 0
  "leave assembble" <- 0
  "Metal rejected temp" <- 0.0 ("Metal rejected")
  "Plastic rejection temp" <- 0.0 ("Plastic rejection temp")
  "Final Assembly" <- 0
  "temp." <- 0
  "Final Metal" <- 0.0 ("final metal")
  "Final Plastic" <- 0.0 ("Final Plastic")
  "Temp.1" <- 0
  "Temp.1 2" <- 0
  "Asem" <- 0
